vi "MainANN_NEW.vi"() -> ()   [LabVIEW 2020]
uses:
  Global Variables/Trainning Done.vi
  Global Variables/Training_Status.vi
  <vilib>/rvi/interface/nirviMethod/nirviMethod.xnode
  <vilib>/rvi/errors/niLvFpgaMergeErrorWithErrorCode.vi
  <vilib>/FPGAPlugInAG/Dynamic/niLvFpga_WriteFifo_Dynamic.vi
  <vilib>/FPGAPlugInAG/Dynamic/niLvFpga_ReadFifo_Dynamic.vi
panel:
  out "Acc":dbl
  in  "?":sgl[](array[numeric])
  out "Classification":sgl[](array[numeric])
  out "Classification Input Layer":sgl[](array[numeric])
  out "trainingRecieved":bool
  in  "Mode":i32
  out "Training Classification":sgl[](array[numeric])
  out "Reading Weights Error":errorcluster
  out "Queue empty":bool
  out "Received Weights and Biases":bool
  in  "Ready to Send":bool
  in  "Read Queue":bool=TRUE
  # "REMARK"
  # "To obtain the Weights the FPGA code has \nto be compiled first! Since the FIFO is flushed, \nimportant when running the logging VI."
  # "Training Data"
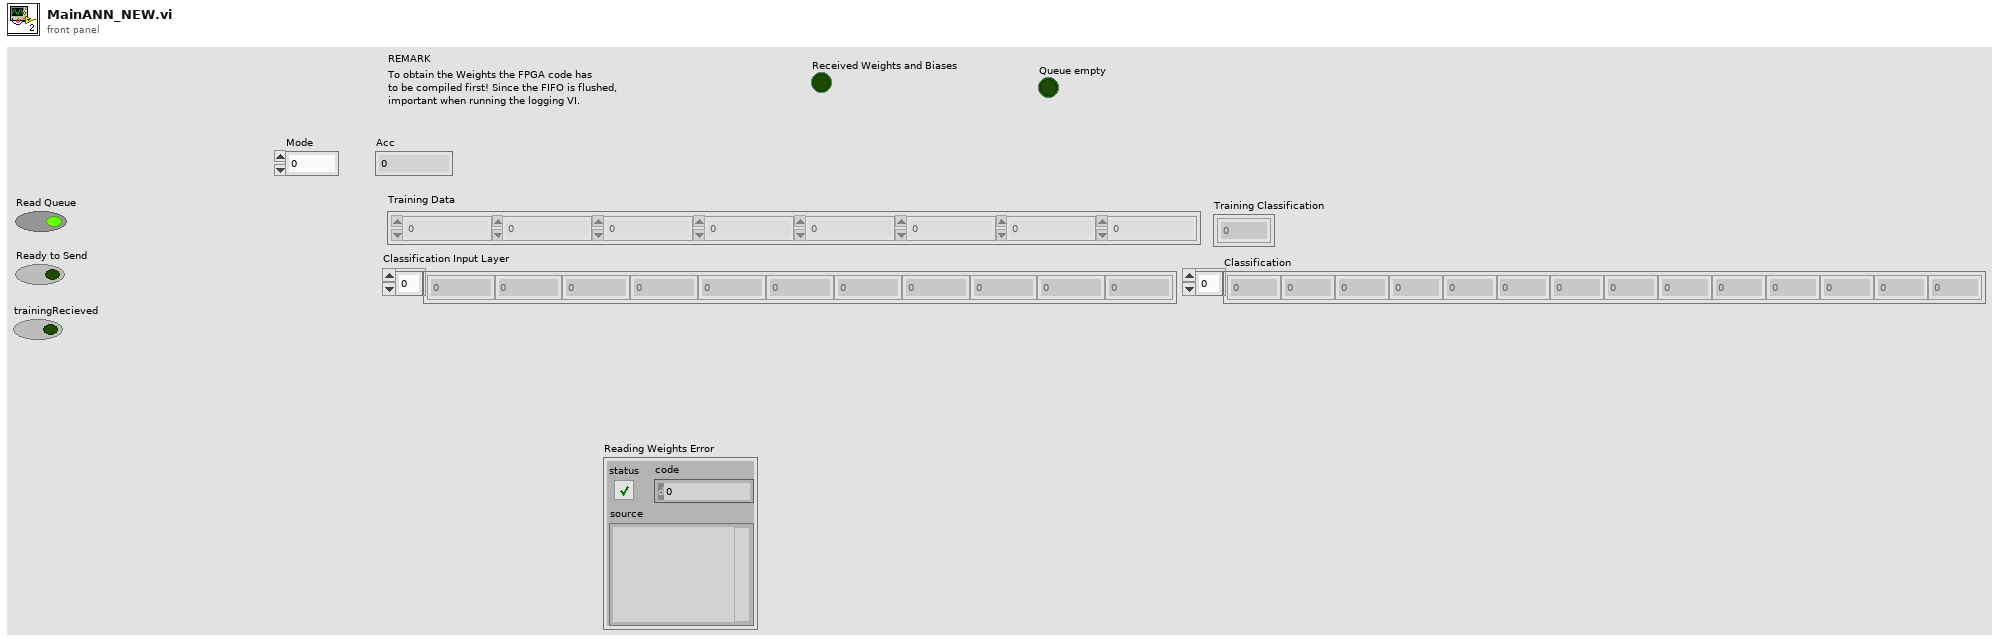
[diagram p1: front panel]
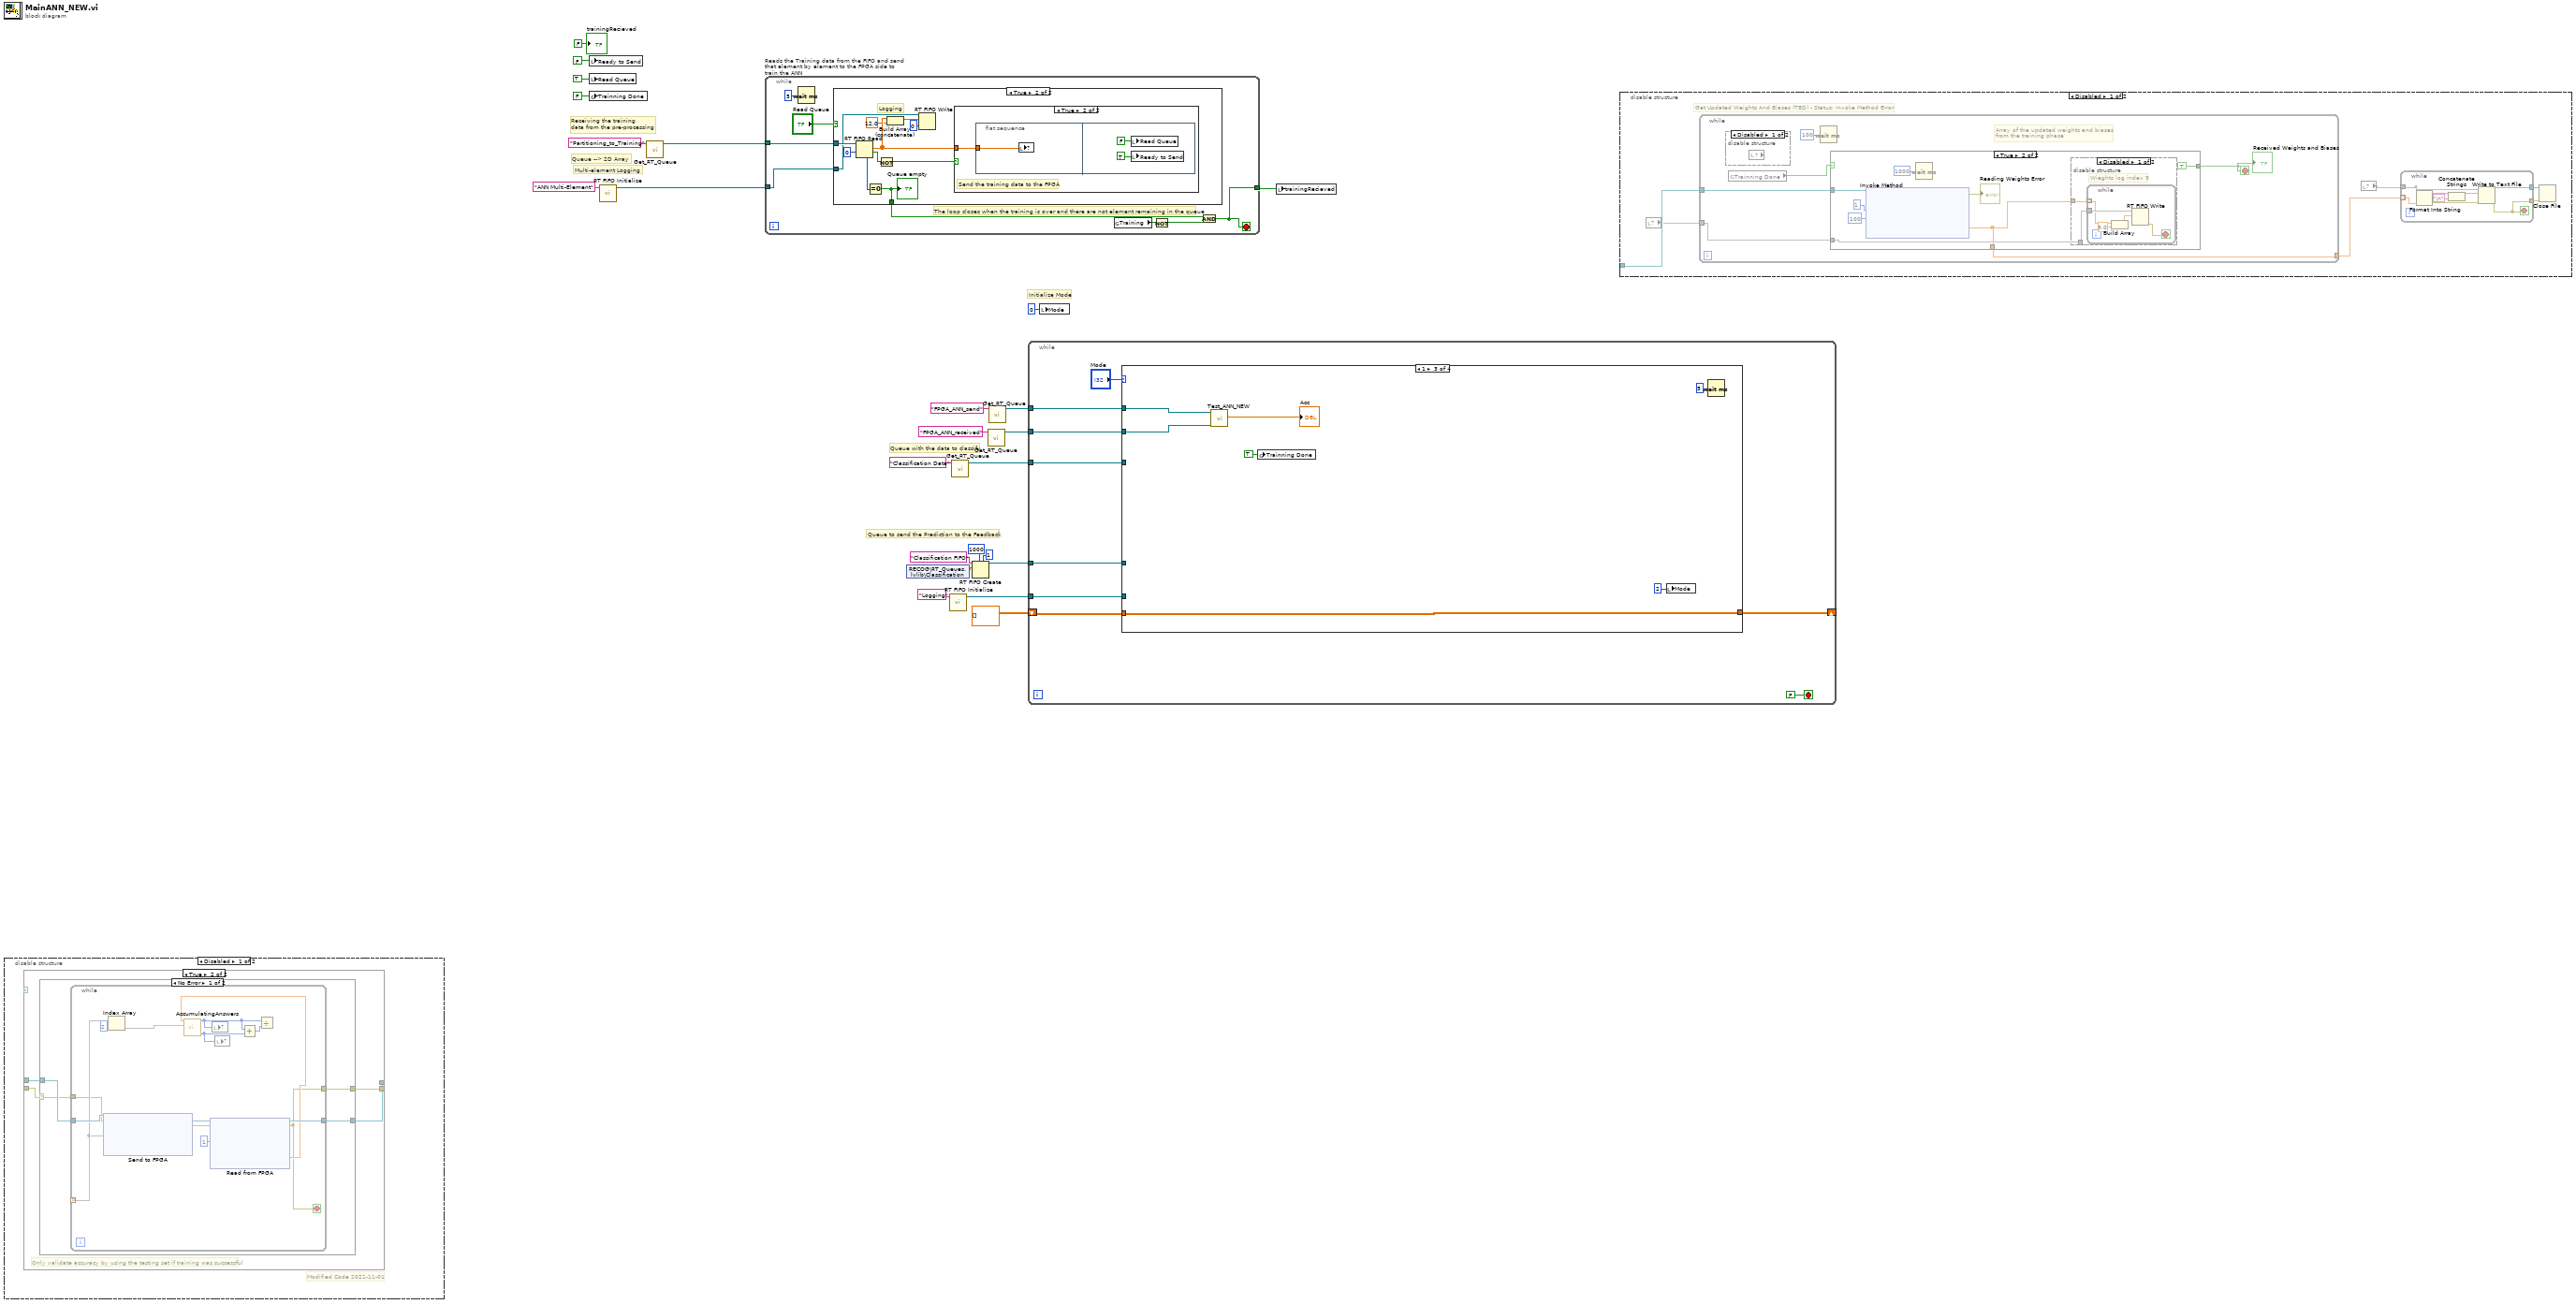
[diagram p0: block diagram]
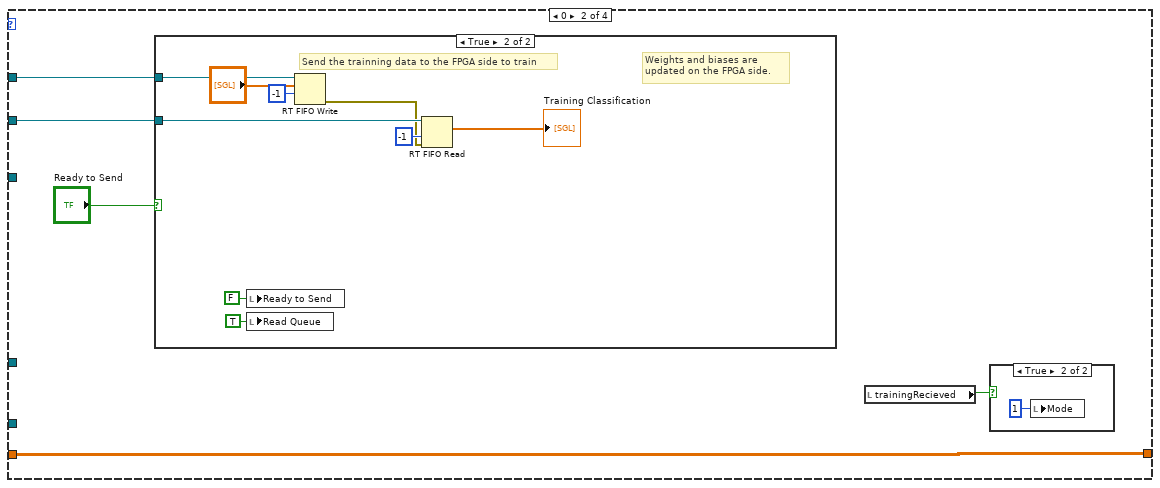
[diagram p3: hidden frame]
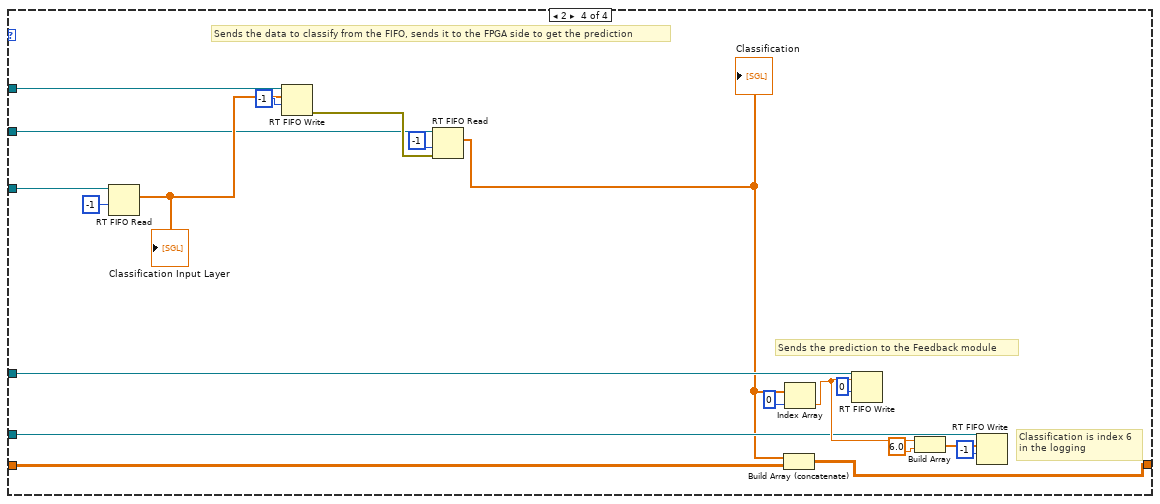
[diagram p6: hidden frame]
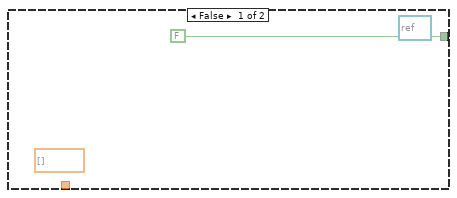
[diagram p8: hidden frame]
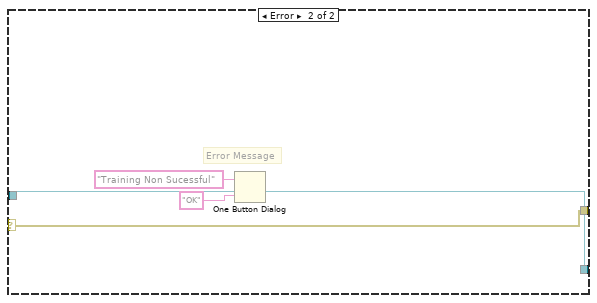
[diagram p12: hidden frame]
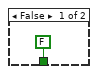
[diagram p14: hidden frame]
diagram:
  # "Initialize Mode"
  # "Queue with the data to classify"
  # "Queue to send the Prediction to the Feedback"
  # "Multi-element Logging"
  # "Receiving the training\ndata from the pre-processing"
  # "Queue --> 2D Array"
  n1 = disable-structure shown="Disabled" {
    frame Disabled {
      # "Modified Code 2021-11-01"
      n2 = case shown="True" {
        selector: _ -> [_ _]
        tunnel: [w26 w31] -> w25
        tunnel: _ -> [w26 w30]
        tunnel: _ -> [w27 w28]
        tunnel: [w27 w29] -> _
        frame False {
        }
        frame True {
          # "Only validate accuracy by using the testing set if training was successful"
          n3 = case shown="No Error" w28 {
            selector: w28 -> [w32 w56]
            tunnel: [w36 w57] -> w31
            tunnel: w30 -> [w35 w57]
            tunnel: [w33 w56] -> w29
            frame No Error {
              n4 = while {
                tunnel: [w40] -> w34 mode=indexing
                tunnel: [w37] -> w33
                tunnel: w32 -> [w38]
                tunnel: w35 -> [w43]
                tunnel: [w47] -> w36
                stop <- w37 stop-if-true
                n5 = xnode "Send to FPGA"("FPGA VI Reference In"=w43, "error in"=w38, "Data"=w40) -> ("FPGA VI Reference Out"=w44:refnum<k20>, "error out"=w45:errorcluster)  [unwired: 1 in, 1 out]
                n6 = Index Array(array=w40, index=2) -> (element=w39)
                n7 = xnode "Read from FPGA"("FPGA VI Reference In"=w44, "error in"=w45, "Number of Elements"=u32 1) -> ("FPGA VI Reference Out"=w47:refnum<k20>, "error out"=w37:errorcluster, "Data"=w46:sgl[])  [unwired: 1 in, 1 out]
                n8 = call "AccumulatingAnswers.vi"("Label"=w39, "Output"=w46) -> (0:"wrong"=w48:i32, 3:"right"=w49:i32, 8:"wrong"=w50:i32, 9:"right"=w51:i32)  [unwired: 6 in]
                n9 = local write item#-1(w49) -> ()
                n10 = local write item#-1(w48) -> ()
                n11 = Add(x=w49, y=w48) -> (x+y=w53:i32)
                n12 = Divide(x=w49, y=w53) -> (x/y=w52:dbl)
              }
            }
            frame Error {
              # "Error Message"
              n13 = One Button Dialog(message="Training Non Sucessful", button name ("OK")="OK") -> ()  [unwired: 1 out]
            }
          }
        }
      }
    }
    frame Enabled {
    }
  }
  n14 = local write "Ready to Send"(FALSE ("Ready to Send")) -> ()
  n15 = local write "Read Queue"(TRUE ("Read Queue")) -> ()
  n16 = global write "Trainning Done.vi" "Trainning Done"(FALSE ("Trainning Done")) -> ()
  n17 = call "RT FIFO Initialize.vi"("name (unnamed)"="ANN Multi-Element") -> ("rt fifo"=w18:refnum<k33>)  [unwired: 9 in, 1 out]
  n18 = call "Get_RT_Queue.vi"("String"="Partitioning_to_Training") -> ("rt fifo single"=w23:refnum<k33>)  [unwired: 8 in, 2 out]
  n19 = while "Reads the Training data from the FIFO and send that element by element to the FPGA side to train the ANN" {
    tunnel: w23 -> [w63]
    tunnel: [w62] -> w16
    tunnel: w18 -> [w58]
    stop <- w62 stop-if-true
    # "The loop closes when the training is over and there are not element remaining in the queue"
    n20 = Wait (ms)(milliseconds to wait=u32 5) -> ()  [unwired: 1 out]
    n21 = case shown="True" "Read Queue" {
      tunnel: w63 -> [_ w75]
      tunnel: [FALSE w72] -> w61
      tunnel: w58 -> [_ w71]
      frame False {
      }
      frame True {
        # "Logging"
        n22 = RT FIFO Read(0:w75, 2:0 ("timeout in ms (0)")) -> (7:w74:u32, 9:w70:sgl[], 10:w77:bool)  [unwired: 2 in, 2 out]
        n23 = Equal To 0?(x=w74) -> (x = 0?=w72:bool)
        "Queue empty" <- w72
        n24 = Not(x=w77) -> (.not. x?=w76:bool)
        n25 = Build Array (concatenate)(w70, 12.0) -> (w68:dbl[])
        n26 = RT FIFO Write(0:w71, 1:w68, 2:0 ("timeout in ms (0)")) -> ()  [unwired: 2 in, 4 out]
        n27 = case shown="True" w76 {
          tunnel: w70 -> [_ w78]
          frame False {
          }
          frame True {
            # "Send the training data to the FPGA"
            n28 = flat-sequence {
              tunnel: w78 -> [w79]
              frame #0 {
                n29 = local write item#10(w79) -> ()
              }
              frame #1 {
                n30 = local write "Read Queue"(FALSE ("Read Queue")) -> ()
                n31 = local write "Ready to Send"(TRUE ("Send Array")) -> ()
              }
            }
          }
        }
      }
    }
    n32 = global read "Training_Status.vi" "Training"() -> (w60:bool)
    n33 = Not(x=w60) -> (.not. x?=w59:bool)
    n34 = And(x=w61, y=w59) -> (x .and. y?=w62:bool)
  }
  n35 = shared-variable "RECOG\\RT_Queues.lvlib\\Classification"() -> (w13:dbl)  [unwired: 1 in, 1 out]
  n36 = call "RT FIFO Initialize.vi"("name (unnamed)"="Logging") -> ("rt fifo"=w9:refnum<k33>)  [unwired: 9 in, 1 out]
  n37 = call "Get_RT_Queue.vi"("String"="Classification Data") -> ("rt fifo single"=w7:refnum<k33>)  [unwired: 8 in, 2 out]
  n38 = RT FIFO Create(0:"Classification FIFO" ("name (unnamed)"), 1:w13, 4:u32 1000 ("size (10)"), 6:u32 1 ("elements in array (1)")) -> (8:w8:refnum<k33>)  [unwired: 4 in, 2 out]
  n39 = call "Get_RT_Queue.vi"("String"="FPGA_ANN_received") -> ("rt fifo single"=w1:refnum<k33>)  [unwired: 8 in, 2 out]
  n40 = call "Get_RT_Queue.vi"("String"="FPGA_ANN_send") -> ("rt fifo single"=w2:refnum<k33>)  [unwired: 8 in, 2 out]
  n41 = while {
    tunnel: w9 -> [w89]
    tunnel: w8 -> [w88]
    tunnel: w7 -> [w87]
    shift-right: [w85] -> _
    shift-left: sgl[][] [] -> [w84]
    tunnel: w2 -> [w83]
    tunnel: w1 -> [w82]
    stop <- FALSE stop-if-true
    n42 = case shown="1" "Mode" {
      tunnel: w89 -> [_ _ _ w126]
      tunnel: w88 -> [_ _ _ w125]
      tunnel: w84 -> [w91 w96 w113 w124]
      tunnel: [w91 w96 w113 w123] -> w85
      tunnel: w87 -> [_ _ _ w121]
      tunnel: w83 -> [_ w93 w109 w117]
      tunnel: w82 -> [_ w92 w108 w115]
      frame Default {
      }
      frame 0 {
        n43 = case shown="True" "Ready to Send" {
          tunnel: w93 -> [_ w104]
          tunnel: w92 -> [_ w101]
          frame False {
          }
          frame True {
            # "Send the trainning data to the FPGA side to train"
            # "Weights and biases are \nupdated on the FPGA side."
            n44 = local write "Ready to Send"(FALSE ("Ready to Send")) -> ()
            n45 = local write "Read Queue"(TRUE ("Read Queue")) -> ()
            n46 = RT FIFO Write(0:w104, 1:"?", 2:-1 ("timeout in ms (0)")) -> (11:w98:errorcluster)  [unwired: 2 in, 3 out]
            n47 = RT FIFO Read(0:w101, 2:-1 ("timeout in ms (0)"), 3:w98) -> (9:→"Training Classification":sgl[])  [unwired: 1 in, 4 out]
          }
        }
        n48 = local read "trainingRecieved"() -> (w94:bool)
        n49 = case shown="True" w94 {
          frame False {
          }
          frame True {
            n50 = local write "Mode"(1 ("Mode")) -> ()
          }
        }
      }
      frame 1 {
        n51 = call "Test_ANN_NEW.vi"("rt fifo READ"=w108, "rt fifo SEND"=w109) -> ("Acc"=→"Acc":dbl)  [unwired: 9 in]
        n52 = global write "Trainning Done.vi" "Trainning Done"(TRUE ("Trainning Done")) -> ()
        n53 = local write "Mode"(2 ("Mode")) -> ()
        n54 = Wait (ms)(milliseconds to wait=u32 5) -> ()  [unwired: 1 out]
      }
      frame 2 {
        # "Classification is index 6\nin the logging"
        # "Sends the prediction to the Feedback module"
        # "Sends the data to classify from the FIFO, sends it to the FPGA side to get the prediction"
        n55 = RT FIFO Read(0:w121, 2:-1 ("timeout in ms (0)")) -> (9:w116:sgl[])  [unwired: 2 in, 4 out]
        "Classification Input Layer" <- w116
        n56 = RT FIFO Write(0:w117, 1:w116, 2:-1 ("timeout in ms (0)")) -> (11:w118:errorcluster)  [unwired: 2 in, 3 out]
        n57 = RT FIFO Read(0:w115, 2:-1 ("timeout in ms (0)"), 3:w118) -> (9:w114:sgl[])  [unwired: 1 in, 4 out]
        "Classification" <- w114
        n58 = Build Array (concatenate)(w114, w124) -> (w123:sgl[][])
        n59 = Index Array(array=w114, index=0) -> (element=w131:sgl)
        n60 = RT FIFO Write(0:w125, 1:w131, 2:0 ("timeout in ms (0)")) -> ()  [unwired: 2 in, 4 out]
        n61 = Build Array(w131, sgl 6.0 ("element")) -> (w129:sgl[])
        n62 = RT FIFO Write(0:w126, 1:w129, 2:-1 ("timeout in ms (0)")) -> ()  [unwired: 2 in, 4 out]
      }
    }
  }
  n63 = local write "Mode"(0 ("Mode")) -> ()
  n64 = local write "trainingRecieved"(w16) -> ()
  n65 = disable-structure shown="Disabled" {
    disable-tunnel: _ -> [w138 _]
    frame Disabled {
      # "Get Updated Weights And Biases (TBD) - Status: Invoke Method Error"
      n66 = local read item#-1() -> (w137)
      n67 = while {
        tunnel: w138 -> [w151]
        tunnel: w137 -> [w149]
        tunnel: [w147] -> w133
        stop <- w150 stop-if-true
        # "Array of the updated weights and biases \nfrom the training phase"
        n68 = disable-structure shown="Disabled" {
          frame Disabled {
            n69 = local read item#-1() -> ()  [unwired: 1 out]
          }
          frame Enabled {
          }
        }
        n70 = global read "Trainning Done.vi" "Trainning Done"() -> (w148:bool)
        n71 = Wait (ms)(milliseconds to wait=u32 100) -> ()  [unwired: 1 out]
        n72 = case shown="True" w148 {
          tunnel: w151 -> [_ w161]
          tunnel: [FALSE TRUE] -> w150
          tunnel: w149 -> [_ w157]
          tunnel: [_ w154] -> w147
          frame False {
            (unwired) sgl[] [] ("Data")
            (unwired) refnum<k20> refnum ("FPGA VI Reference Out")
          }
          frame True {
            n73 = xnode "Invoke Method"("FPGA VI Reference In"=w161, "Number of Elements"=u32 1, "Timeout (ms)"=100) -> ("error out"=→"Reading Weights Error":errorcluster, "Data"=w154:sgl[])  [unwired: 1 in, 2 out]
            n74 = Wait (ms)(milliseconds to wait=u32 1000) -> ()  [unwired: 1 out]
            n75 = disable-structure shown="Disabled" {
              disable-tunnel: w157 -> [w163 _]
              disable-tunnel: w154 -> [w162 _]
              frame Disabled {
                # "Wieghts log index 9"
                n76 = while {
                  tunnel: w163 -> [w168]
                  tunnel: w162 -> [w167] mode=indexing
                  stop <- w164 stop-if-true
                  n77 = Build Array(w167, sgl 9.0 ("element")) -> (w165:sgl[])
                  n78 = RT FIFO Write(0:w168, 1:w165) -> (11:w164:errorcluster)  [unwired: 3 in, 3 out]
                }
              }
              frame Enabled {
              }
            }
          }
        }
        "Received Weights and Biases" <- w150
      }
      n79 = local read item#-1() -> (w134)
      n80 = while {
        tunnel: [w146] -> _
        tunnel: w134 -> [w146]
        tunnel: w133 -> [w145] mode=indexing
        tunnel: [w141] -> w135
        tunnel: [w139] -> w136
        stop <- w139 stop-if-true
        n81 = Format Into String(w145) -> (resulting string=w144:string, error out=w140:errorcluster)  [unwired: 3 in]
        n82 = Concatenate Strings(w144, "\n") -> (w143:string)
        n83 = Write to Text File(file (use dialog)=w146, text=w143, error in=w140) -> (refnum out=w141:refnum<file>, error out=w139:errorcluster)  [unwired: 1 in, 1 out]
      }
      n84 = Close File(refnum=w135, error in=w136) -> ()  [unwired: 2 out]
    }
    frame Enabled {
    }
  }
  "trainingRecieved" <- FALSE ("trainingRecieved")
